vi "Interpolation (Control - Window Init Mem) Test.vi"() -> ()   [LabVIEW 2014]
uses:
  <vilib>/FPGAPlugInAG/sbRIO-9636/niLvFpga_Open_sbRIO-9636.vi
  <vilib>/rvi/interface/common/dynamic/niFpgaDynamicAddResources.vi
  <vilib>/Utility/error.llb/Error Cluster From Error Code.vi
  <vilib>/rvi/errors/niLvFpgaAdjustHostInterfaceError.vi
  <vilib>/rvi/interface/common/niFpgaWaitOnOcc.vi
  <vilib>/FPGAPlugInAG/Dynamic/niLvFpga_Run_Dynamic.vi
  <vilib>/FPGAPlugInAG/Dynamic/niLvFpga_Abort_Dynamic.vi
  <vilib>/FPGAPlugInAG/Dynamic/niLvFpga_Close_Dynamic.vi
  <vilib>/rvi/interface/nirviOpenFPGA/nirviOpenFPGA.xnode
  FPGA Bitfiles/LaserDistanceSen_FPGATarget_FFTnoclk_fKZd8IB86m8.lvbitx
  FPGA Target/Test VIs/FFT no clk.vi
  <vilib>/rvi/interface/nirviReadWriteControl/nirviReadWriteControl.xnode
  <vilib>/rvi/interface/nirviMethod/nirviMethod.xnode
  <vilib>/rvi/interface/nirviCloseFPGA/nirviCloseFPGA.xnode
  <vilib>/FPGAPlugInAG/Dynamic/niLvFpga_ConfigureFifo_Dynamic.vi
  <vilib>/rvi/errors/niLvFpgaMergeErrorWithErrorCode.vi
  <vilib>/FPGAPlugInAG/Dynamic/niLvFpga_StartFifo_Dynamic.vi
  NiFpgaLv.dll
  <vilib>/rvi/interface/Simulation/niFpgaSimulationCallBeginRW.vi
panel:
  out "Distance":dbl
  out "Ftone+":dbl
  out "Ftone-":dbl
  in  "Windowing":T1(ring)=enum."Hamming"
  in  "first bin":i32=10
  in  "last bin":i32=255
  in  "lower limit 2":u32(slide)=677 scale=625.0..737.0
  in  "lower limit 1":u32(slide)=59 scale=0.0..112.0
  out "Detected Frequency Tone - (Hz)":dbl
  in  "stop":bool
  out "Max Bin":i32
  out "Max Amp":dbl format="%.2f"
  out "Prev Bin":i32
  out "Next Bin":i32
  out "Prev Amp":dbl format="%.2f"
  out "Next Amp":dbl format="%.2f"
  out "Interpolated Bin":dbl
  in  "Interpolation Method":T2(ring)
  # "OFFLINE parameters"
  # "ONLINE parameter"
  # "Max Detection FFT bin range"
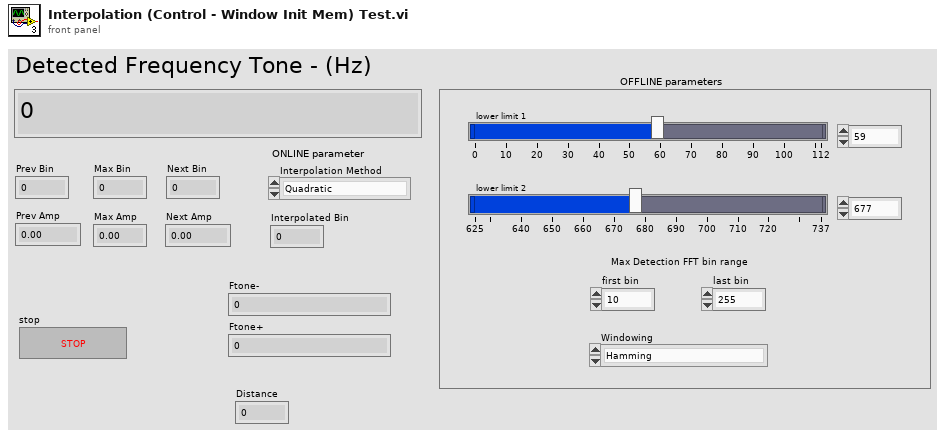
[diagram p1: front panel]
types:
  T1 = enum16{"None", "Hanning", "Hamming", "Blackman", "Blackman-Harris"}
  T2 = enum16{"Quadratic", "McLeodd", "Barycentric", "Jain"}
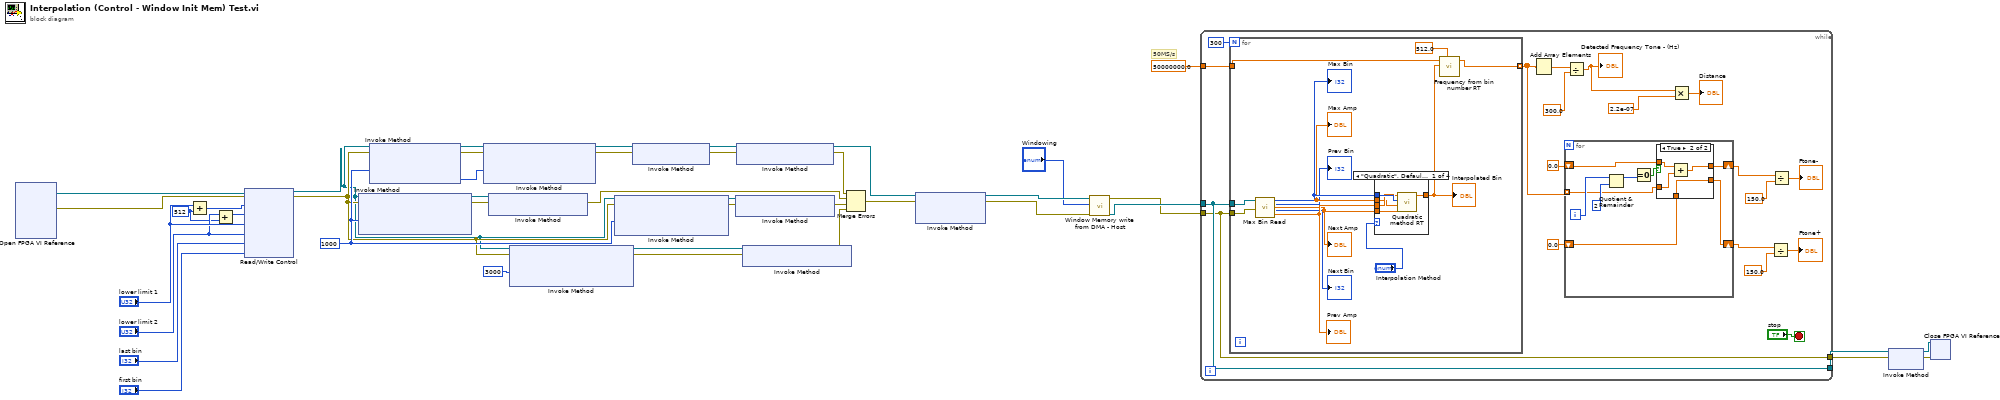
[diagram p0: block diagram]
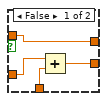
[diagram p2: hidden frame]
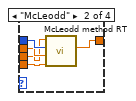
[diagram p3: hidden frame]
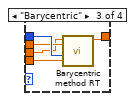
[diagram p4: hidden frame]
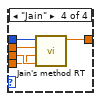
[diagram p5: hidden frame]
diagram:
  w11 = u32 512 ("y")
  w30 = u32 1000 ("Requested Depth")
  # "50MS/s"
  n1 = xnode "Open FPGA VI Reference"() -> ("FPGA VI Reference Out"=w8:refnum<k20>, "error out"=w7:errorcluster)  [unwired: 2 in]
  n2 = Add(x="lower limit 1", y=w11) -> (x+y=w15:u32)
  n3 = Add(x="lower limit 2", y=w11) -> (x+y=w13:u32)
  n4 = xnode "Read/Write Control"("FPGA VI Reference In"=w8, "error in"=w7, "upper limit 1"=w15, "upper limit 2"=w13, "lower limit 1"="lower limit 1", "lower limit 2"="lower limit 2", "last bin"="last bin", "first bin"="first bin") -> ("FPGA VI Reference Out"=w9:refnum<k20>, "error out"=w10:errorcluster)
  n5 = xnode "Invoke Method"("FPGA VI Reference In"=w9, "error in"=w10, "Requested Depth"=w30) -> ("FPGA VI Reference Out"=w31:refnum<k20>, "error out"=w32:errorcluster)  [unwired: 1 out]
  n6 = xnode "Invoke Method"("FPGA VI Reference In"=w9, "error in"=w10, "Requested Depth"=w30) -> ("FPGA VI Reference Out"=w42:refnum<k20>, "error out"=w41:errorcluster, "Actual Depth"=w40:u32)
  n7 = xnode "Invoke Method"("FPGA VI Reference In"=w42, "error in"=w41, "Requested Depth"=w40) -> ("FPGA VI Reference Out"=w39:refnum<k20>, "error out"=w38:errorcluster)  [unwired: 1 out]
  n8 = xnode "Invoke Method"("FPGA VI Reference In"=w31, "error in"=w32) -> ("error out"=w34:errorcluster)  [unwired: 1 out]
  n9 = xnode "Invoke Method"("FPGA VI Reference In"=w9, "error in"=w10, "Requested Depth"=u32 3000) -> ("FPGA VI Reference Out"=w27:refnum<k20>, "error out"=w26:errorcluster)  [unwired: 1 out]
  n10 = xnode "Invoke Method"("FPGA VI Reference In"=w9, "error in"=w10, "Requested Depth"=w30) -> ("FPGA VI Reference Out"=w29:refnum<k20>, "error out"=w28:errorcluster)  [unwired: 1 out]
  n11 = xnode "Invoke Method"("FPGA VI Reference In"=w39, "error in"=w38) -> ("FPGA VI Reference Out"=w37:refnum<k20>, "error out"=w36:errorcluster)
  n12 = xnode "Invoke Method"("FPGA VI Reference In"=w29, "error in"=w28) -> ("error out"=w33:errorcluster)  [unwired: 1 out]
  n13 = xnode "Invoke Method"("FPGA VI Reference In"=w37, "error in"=w36) -> ("FPGA VI Reference Out"=w5:refnum<k20>, "error out"=w35:errorcluster)
  n14 = xnode "Invoke Method"("FPGA VI Reference In"=w27, "error in"=w26) -> ("error out"=w24:errorcluster)  [unwired: 1 out]
  n15 = Merge Errors(w35, w34, w33, w24) -> (w6:errorcluster)
  n16 = xnode "Invoke Method"("FPGA VI Reference In"=w5, "error in"=w6) -> ("FPGA VI Reference Out"=w21:refnum<k20>, "error out"=w22:errorcluster)  [unwired: 1 in]
  n17 = call "Window Memory write from DMA - Host.vi"("error in"=w22, "Enum"="Windowing", "FPGA VI Reference In"=w21) -> ("FPGA VI Reference Out"=w19:refnum<k20>, "error out"=w18:errorcluster)  [unwired: 5 in, 2 out]
  n18 = while {
    tunnel: 50000000.0 ("Sample Rate (S/s)") -> [w59]
    tunnel: w19 -> [w60]
    tunnel: w18 -> [w46]
    tunnel: [w60] -> w2
    tunnel: [w46] -> w3
    stop <- "stop" stop-if-true
    n19 = for {
      N: 300 -> [_]
      tunnel: w60 -> [w83]
      tunnel: w46 -> [w82]
      tunnel: w59 -> [w81]
      tunnel: [w79] -> w51 mode=indexing
      n20 = call "Max Bin Read.vi"("FPGA VI Reference In"=w83, "error in"=w82) -> ("Max Bin"=w91:i32, "Max Amp"=w90:dbl, "Prev Bin"=→"Prev Bin":i32, "Next Amp"=w87:dbl, "Next Bin"=→"Next Bin":i32, "Prev Amp"=w88:dbl)  [unwired: 12 in]
      "Max Bin" <- w91
      "Max Amp" <- w90
      "Prev Amp" <- w88
      "Next Amp" <- w87
      n21 = case shown="\"Quadratic\", Default" "Interpolation Method" {
        tunnel: w91 -> [w95 w100 w105 w110]
        tunnel: w90 -> [w92 w99 w104 w109]
        tunnel: w88 -> [w93 w98 w103 w108]
        tunnel: w87 -> [w94 w97 w102 w107]
        tunnel: [w96 w101 w106 w111] -> w80
        frame "Quadratic", Default {
          n22 = call "Quadratic method RT.vi"("Next Amplitude"=w94, "Max Amplitude"=w92, "Max bin"=w95, "Prev Amplitude"=w93) -> ("Bin"=w96:dbl)  [unwired: 7 in]
        }
        frame "McLeodd" {
          n23 = call "McLeodd method RT.vi"("Next Amp"=w97, "Max Amp"=w99, "Max Bin"=w100, "Prev Amp"=w98) -> ("Bin"=w101:dbl)  [unwired: 7 in]
        }
        frame "Barycentric" {
          n24 = call "Barycentric method RT.vi"("Next Amp"=w102, "Max Bin"=w105, "Max Amp"=w104, "Prev Amp"=w103) -> ("Bin"=w106:dbl)  [unwired: 7 in]
        }
        frame "Jain" {
          n25 = call "Jain's method RT.vi"("Prev Amp"=w108, "Next Amp"=w107, "Max Amp"=w109, "Max Bin"=w110) -> ("Bin"=w111:dbl)  [unwired: 7 in]
        }
      }
      "Interpolated Bin" <- w80
      n26 = call "Frequency from bin number RT.vi"("FFT size"=512.0, "Bin number"=w80, "Sample Rate (S/s)"=w81) -> ("Detected Frequency (Hz)"=w79:dbl)  [unwired: 8 in]
    }
    n27 = Add Array Elements(numeric array=w51) -> (sum=w58:dbl)
    n28 = for {
      tunnel: w51 -> [w65] mode=indexing
      shift-right: [w64] -> w54
      shift-left: 0.0 -> [w66]
      shift-right: [w62] -> w47
      shift-left: 0.0 -> [w63]
      i -> [w70]
      n29 = Quotient & Remainder(x=w70, y=2) -> (x-y*floor(x/y)=w68:i32)  [unwired: 1 out]
      n30 = Equal To 0?(x=w68) -> (x = 0?=w67:bool)
      n31 = case shown="True" w67 {
        tunnel: w66 -> [w74 w78]
        tunnel: w65 -> [w73 w77]
        tunnel: [w74 w76] -> w64
        tunnel: w63 -> [w72 w75]
        tunnel: [w71 w75] -> w62
        frame False {
          n32 = Add(x=w73, y=w72) -> (x+y=w71:dbl)
        }
        frame True {
          n33 = Add(x=w78, y=w77) -> (x+y=w76:dbl)
        }
      }
    }
    n34 = Divide(x=w58, y=300.0) -> (x/y=w44:dbl)
    "Detected Frequency Tone - (Hz)" <- w44
    n35 = Multiply(x=w44, y=2.2e-07) -> (x*y=→"Distance":dbl)
    n36 = Divide(x=w47, y=150.0) -> (x/y=→"Ftone+":dbl)
    n37 = Divide(x=w54, y=150.0) -> (x/y=→"Ftone-":dbl)
  }
  n38 = xnode "Invoke Method"("FPGA VI Reference In"=w2, "error in"=w3) -> ("FPGA VI Reference Out"=w4:refnum<k20>, "error out"=w20:errorcluster)
  n39 = xnode "Close FPGA VI Reference"("FPGA VI Reference In"=w4, "error in"=w20) -> ()  [unwired: 1 out]
